vi "Peak Detector.vi"(4 "end of data (T)":bool=TRUE, 6 "initialize (T)":bool=TRUE, 8 "peaks/valleys":enum32{"Peaks", "Valleys"}(ring), 9 "width":i32=3 min=3, 10 "threshold":dbl format="%0.2f", 11 "X":dbl[](array[numeric])) -> (0 "error":i32, 1 "2nd Derivatives":dbl[](array[numeric]), 2 "Amplitudes":dbl[](array[numeric]), 3 "Locations":dbl[](array[numeric]), 5 "# found":i32)   [LabVIEW 2011, in "NI_AAL_SigProc.lvlib"]
doc: "Finds the location, amplitude, and second derivative of peaks or valleys in the input signal."
uses:
  NI_AAL_SigProc.lvlib
  lvanlys.dll
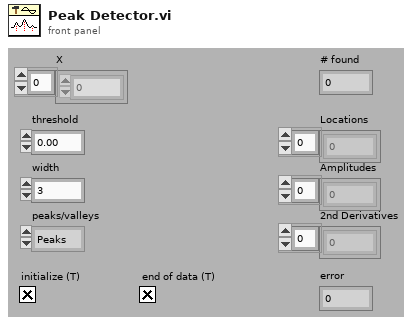
[diagram p1: front panel]
types:
  T1 = cluster{"Span":i32, "Index":i32, "NHistoryPts":i32, "Len":i32, "PrevSign":i32, "unused":i32, "RinvQt (pointer)":u32, "FitBuffer (pointer)":u32, "History (pointer)":u32, "PrevCoeff (pointer)":u32, "Data (pointer)":u32, "slack for RinvQt":u32, "slack for FitBuffer":u32, "slack for History":u32, "slack for PrevCoeff":u32, "slack for Data":u32}
  T2 = cluster{"X":dbl[], "threshold":dbl, "Span":i32, "peaks/valleys":enum32{"Peaks", "Valleys"}, "Array Constant":dbl[], "Array Constant":dbl[], "Array Constant":dbl[], i32, i32}
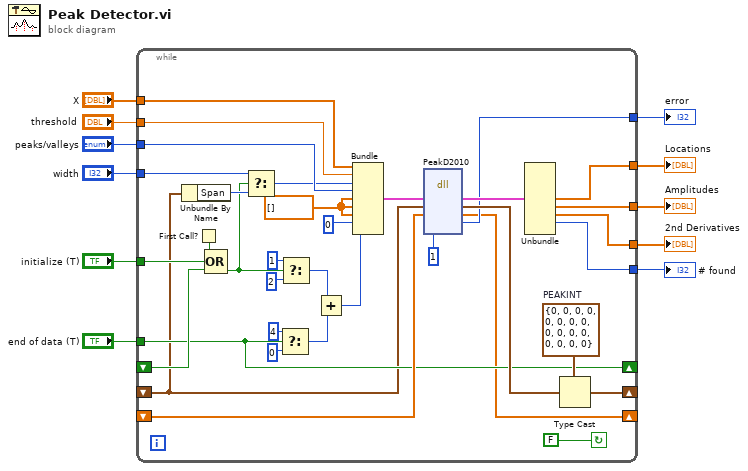
[diagram p0: block diagram]
diagram:
  n1 = while {
    shift-left: _ -> [w32]
    shift-right: [w19] -> _
    shift-left: _ -> [w26]
    shift-right: [w20] -> _
    shift-right: [w28] -> _
    shift-left: _ -> [w35]
    tunnel: "X" -> [w31]
    tunnel: "threshold" -> [w30]
    tunnel: "width" -> [w22]
    tunnel: "peaks/valleys" -> [w29]
    tunnel: "end of data (T)" -> [w28]
    tunnel: "initialize (T)" -> [w27]
    tunnel: [w21] -> w5
    tunnel: [w18] -> w4
    tunnel: [w17] -> w3
    tunnel: [w16] -> w2
    tunnel: [w15] -> w1
    stop <- FALSE continue-if-true
    w36 = T1 {"Span"=0, "Index"=0, "NHistoryPts"=0, "Len"=0, "PrevSign"=0, "unused"=0, "RinvQt (pointer)"=0, "FitBuffer (pointer)"=0, "History (pointer)"=0, "PrevCoeff (pointer)"=0, "Data (pointer)"=0, "slack for RinvQt"=0, "slack for FitBuffer"=0, "slack for History"=0, "slack for PrevCoeff"=0, "slack for Data"=0}  # PEAKINT
    w39 = dbl[] [] ("Array Constant")
    n2 = Unbundle By Name(w26) -> ("Span"=w25:i32)
    n3 = First Call?() -> (First Call?: T/F=w34:bool)
    n4 = Compound Arithmetic op=OR(w34, w27, w35) -> (w24:bool)
    n5 = Select(t=w22, s=w24, f=w25) -> (s? t:f=w23:i32)
    n6 = Select(t=4, s=w28, f=0) -> (s? t:f=w13:i32)
    n7 = Select(t=1, s=w24, f=2) -> (s? t:f=w14:i32)
    n8 = Add(x=w14, y=w13) -> (x+y=w41:i32)
    n9 = Bundle("X"=w31, "threshold"=w30, "Span"=w23, "peaks/valleys"=w29, "Array Constant"=w39, "Array Constant"=w39, "Array Constant"=w39, 0, w41) -> (w33:T2)  [unwired: 1 out]
    n10 = dll-call lib="C:/Program Files/National Instruments/LabVIEW 2011/resource/lvanlys.*" fn="PeakD2010"("PeakApp"=w33, "pPEAKINT"=w26, "SavedData"=w32, "version"=1) -> ("PeakApp"=w40:T2, "pPEAKINT"=w37:T1, "SavedData"=w19:dbl[], "pErr"=w21:i32)  [unwired: 3 in, 5 out]
    n11 = Unbundle(w40) -> ("Array Constant"=w18:dbl[], "Array Constant"=w17:dbl[], "Array Constant"=w16:dbl[], w15:i32)  [unwired: 5 out]
    n12 = Type Cast(type=w36, x=w37) -> (*(type *) &x=w20:T1)
  }
  "Locations" <- w4
  "Amplitudes" <- w3
  "2nd Derivatives" <- w2
  "error" <- w5
  "# found" <- w1
